vi "Set Velocity 2.vi"(0 "Process Variable(x)":dbl=-39665.0, 5 "Current TIme":u32=2704019, 7 "Current Power":dbl=0.3631999999999999, 9 "Setpoint(end)":dbl=39120.0, 11 "Total Distance":dbl=39120.0 format="%#_13g", 12 "Last Time Input":u32=2703907) -> (4 "Coerced Motor power":dbl format="%#_13g", 6 "End Loop?":bool=TRUE, 8 "Non-Coerced Motor Power":dbl, 10 "Last Time Output":u32=2704019)   [LabVIEW 2016]
panel:
  in  "Tick range":dbl=300.0 format="%#_13g"
  in  "Power Constant (power/ms^2) constant":dbl=0.0002 format="%#_13g"
  in  "Robot Barely Moving Power":dbl=0.2 format="%#_13g"
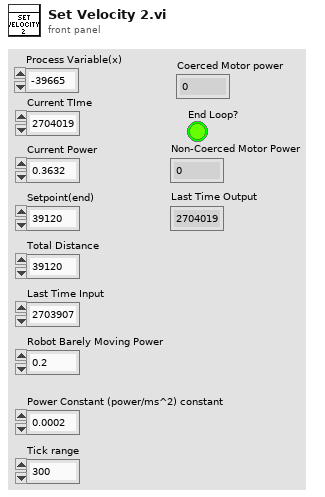
[diagram p1: front panel]
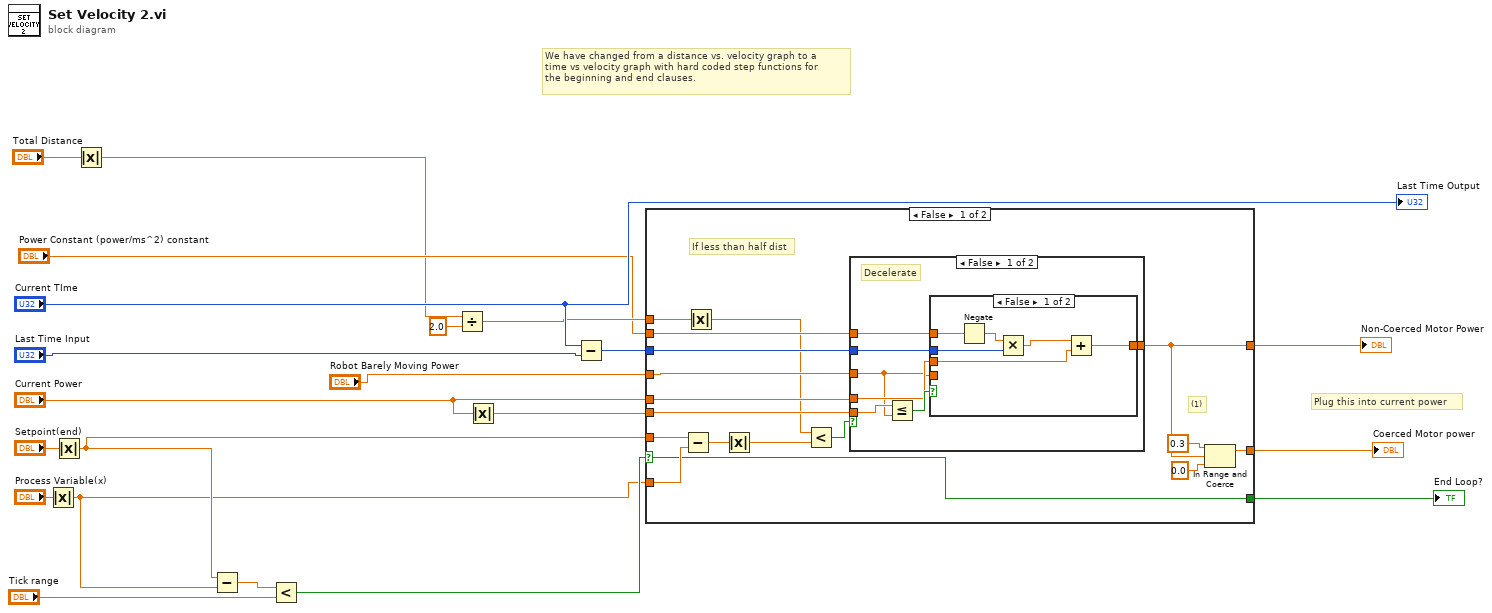
[diagram p0: block diagram]
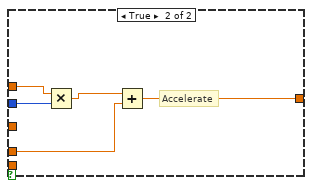
[diagram p3: hidden frame]
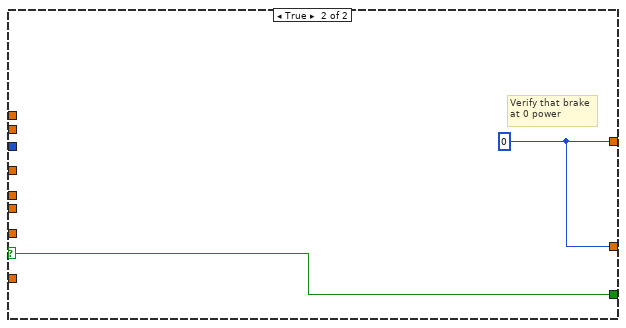
[diagram p4: hidden frame]
diagram:
  # "Plug this into current power"
  # "We have changed from a distance vs. velocity graph to a\ntime vs velocity graph with hard coded step functions for \nthe beginning and end clauses."
  n1 = Absolute Value(x="Process Variable(x)") -> (abs(x)=w1:dbl)
  n2 = Absolute Value(x="Setpoint(end)") -> (abs(x)=w2:dbl)
  n3 = Absolute Value(x="Total Distance") -> (abs(x)=w3:dbl)
  n4 = Subtract(x=w2, y=w1) -> (x-y=w4:dbl)
  n5 = Less?(x=w4, y="Tick range") -> (x < y?=w6:bool)
  n6 = Divide(x=w3, y=2.0) -> (x/y=w13:dbl)
  n7 = Absolute Value(x="Current Power") -> (abs(x)=w12:dbl)
  n8 = Subtract(x="Current TIme", y="Last Time Input") -> (x-y=w18:u32)
  n9 = case shown="False" w6 {
    selector: w6 -> [w33 w59]
    tunnel: w2 -> [w38 _]
    tunnel: w1 -> [w37 _]
    tunnel: [w35 w58] -> w21
    tunnel: [w33 w59] -> w20
    tunnel: w13 -> [w31 _]
    tunnel: "Robot Barely Moving Power" -> [w27 _]
    tunnel: w18 -> [w30 _]
    tunnel: "Current Power" -> [w25 _]
    tunnel: w12 -> [w28 _]
    tunnel: "Power Constant (power/ms^2) constant" -> [w26 _]
    tunnel: [w24 w58] -> w5
    frame False {
      # "(1)"
      # "If less than half dist"
      n10 = Subtract(x=w38, y=w37) -> (x-y=w36:dbl)
      n11 = Absolute Value(x=w31) -> (abs(x)=w23:dbl)
      n12 = Absolute Value(x=w36) -> (abs(x)=w32:dbl)
      n13 = Less?(x=w23, y=w32) -> (x < y?=w29:bool)
      n14 = case shown="False" w29 {
        tunnel: w30 -> [w41 w57]
        tunnel: [w43 w54] -> w24
        tunnel: w27 -> [w39 _]
        tunnel: w28 -> [w45 _]
        tunnel: w26 -> [w42 w56]
        tunnel: w25 -> [w40 w55]
        frame False {
          # "Decelerate"
          n15 = Less Or Equal?(x=w45, y=w39) -> (x <= y?=w44:bool)
          n16 = case shown="False" w44 {
            tunnel: [w47 w52] -> w43
            tunnel: w39 -> [_ w52]
            tunnel: w42 -> [w50 _]
            tunnel: w41 -> [w49 _]
            tunnel: w40 -> [w48 _]
            frame False {
              n17 = Negate(x=w50) -> (-x=w51:dbl)
              n18 = Multiply(x=w51, y=w49) -> (x*y=w46:dbl)
              n19 = Add(x=w46, y=w48) -> (x+y=w47:dbl)
            }
            frame True {
              # "Sets to barely moving power"
            }
          }
        }
        frame True {
          # "Accelerate"
          n20 = Multiply(x=w56, y=w57) -> (x*y=w53:dbl)
          n21 = Add(x=w53, y=w55) -> (x+y=w54:dbl)
        }
      }
      n22 = In Range and Coerce(upper limit=0.3, x=w24, lower limit=0.0) -> (coerced(x)=w35:dbl)  [unwired: 1 out]
    }
    frame True {
      w58 = 0
      # "Verify that brake\nat 0 power"
    }
  }
  "End Loop?" <- w20
  "Coerced Motor power" <- w21
  "Non-Coerced Motor Power" <- w5
  "Last Time Output" <- "Current TIme"
